vi "Encendido de alarmas_temperaturas.vi"() -> ()   [LabVIEW 2013]
panel:
  out "agradable":bool
  out "mayor a 40":bool
  out "ValorTemperatura":dbl
  out "Temperatura":i32(slide) scale=0.0..60.0
  # "temperatura agradable"
  # "encender la alarma cuando la temperatura\nsea mayor a 40 grados"
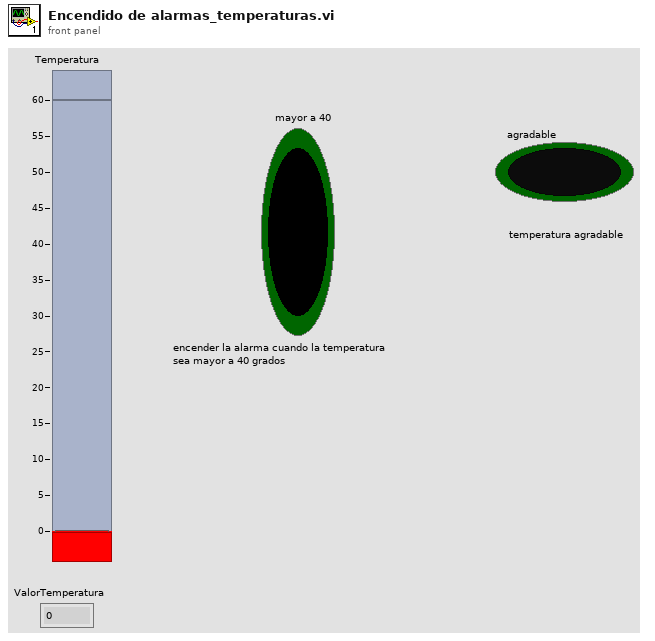
[diagram p1: front panel]
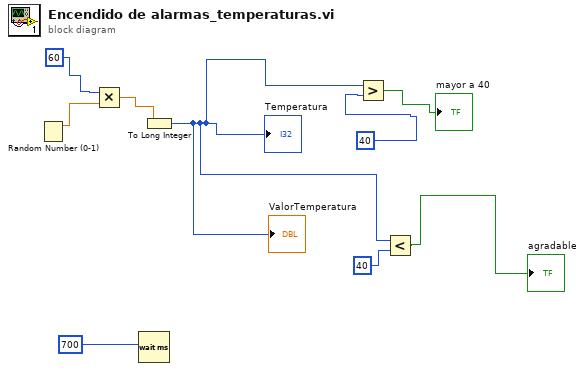
[diagram p0: block diagram]
diagram:
  n1 = Random Number (0-1)() -> (number: 0 to 1=w8:dbl)
  n2 = Multiply(x=60, y=w8) -> (x*y=w7:dbl)
  n3 = Wait (ms)(milliseconds to wait=700) -> ()  [unwired: 1 out]
  n4 = To Long Integer(number=w7) -> (32bit integer=w3:i32)
  "Temperatura" <- w3
  "ValorTemperatura" <- w3
  n5 = Greater?(x=w3, y=40) -> (0:→"mayor a 40":bool)
  n6 = Less?(x=w3, y=40) -> (x < y?=→"agradable":bool)
